vi "ClusterRef_2_DisplayTemplatesRef.vi"(8 "error in (no error)":errorcluster, 11 "Cluster Refnum":refnum<vi>) -> (0 "error out":errorcluster, 3 "Framework Templates":refnum<vi>)   [LabVIEW 2021, in "FakedArray.lvclass"]
uses:
  <resource>/plugins/NIIconEditor/Class/FakedArray/FakedArray.lvclass
panel:
  in  "Framework Templates 2":refnum<vi>
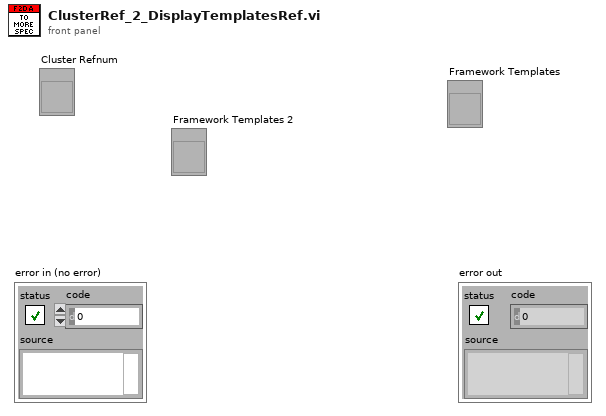
[diagram p1: front panel]
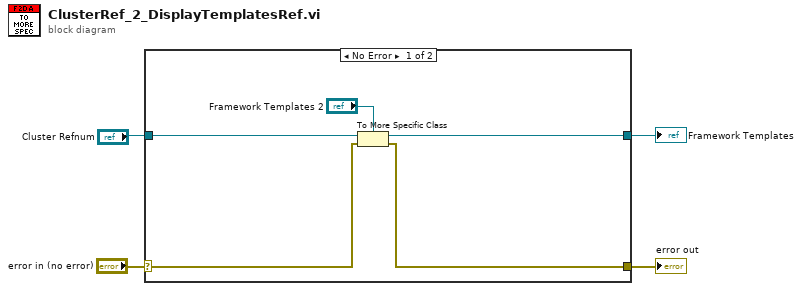
[diagram p0: block diagram]
diagram:
  n1 = case shown="No Error" "error in (no error)" {
    selector: "error in (no error)" -> [w6 w10]
    tunnel: [w5 w10] -> w3
    tunnel: [w8 _] -> w2
    tunnel: "Cluster Refnum" -> [w7 _]
    frame No Error {
      n2 = To More Specific Class(target class="Framework Templates 2", reference=w7, error in=w6) -> (specific class reference=w8:refnum<vi>, error out=w5:errorcluster)
    }
    frame Error {
    }
  }
  "error out" <- w3
  "Framework Templates" <- w2
